vi "Create new scene_3Dpf.vi"(2 "Translation":cluster{"X":sgl, "Y":sgl, "Z":sgl}, 3 "Scale":cluster{"X":sgl, "Y":sgl, "Z":sgl}={"X"=1.0, "Y"=1.0, "Z"=1.0}, 4 "Scene objects array":refnum<vi>[](array[refnum])) -> (0 "Error out":errorcluster, 1 "Scene out":refnum<vi>)   [LabVIEW 2017]
doc: "Use this VI to add an array of scene objects to a new rendering scene (for output to a render window or 3D picture control)."
uses:
  <vilib>/picture/3D Picture Control/Object/Add Object (no reference).vi
  <vilib>/picture/3D Picture Control/Object/Create Object (name).vi
  <vilib>/picture/3D Picture Control/NI_3D Picture Control.lvlib
panel:
  # "PN 03/02/2015"
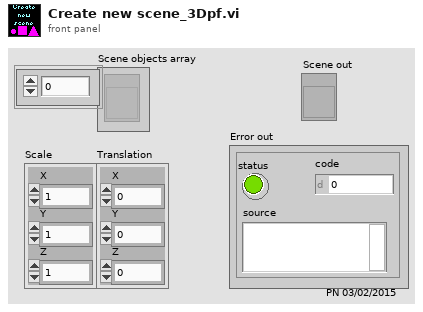
[diagram p1: front panel]
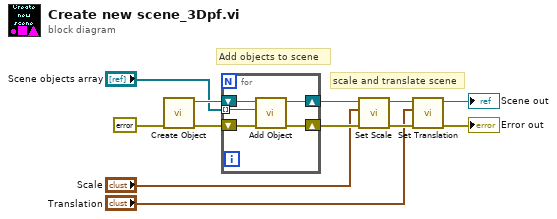
[diagram p0: block diagram]
diagram:
  # "Add objects to scene"
  # "scale and translate scene"
  n1 = call-poly <vilib>:"Create Object.vi"("error in (no error)"=errorcluster {"status"=FALSE, "code"=0, "source"=""}) -> ("error out"=w8:errorcluster, "Scene:New Object"=w9:refnum<vi>)  [unwired: 9 in]
  n2 = for {
    tunnel: "Scene objects array" -> [w17] mode=indexing
    shift-right: [w15] -> w6
    shift-left: w9 -> [w16]
    shift-right: [w13] -> w7
    shift-left: w8 -> [w14]
    n3 = call-poly <vilib>:"Add Object.vi"("error in (no error)"=w14, "New Object In"=w17, "Scene Object In"=w16) -> ("error out"=w13:errorcluster, "Scene Object Out"=w15:refnum<vi>)  [unwired: 7 in]
  }
  n4 = call <vilib>:"Set Scale.vi"("error in (no error)"=w7, "Scale"="Scale", "Scene Object"=w6) -> ("error out"=w11:errorcluster, "Scaled Object"=w10:refnum<vi>)  [unwired: 7 in]
  n5 = call <vilib>:"Set Translation.vi"("error in (no error)"=w11, "Translation"="Translation", "Scene Object"=w10) -> ("error out"=→"Error out":errorcluster, "Translated Object"=→"Scene out":refnum<vi>)  [unwired: 7 in]
